vi "Word Search.vi"() -> ()   [LabVIEW 2020]
panel:
  in  "number of words":i32=300
  in  "Max Word Length":u64=150
  in  "Min Word Length":u64=10
  in  "size (rows, columns)":i32[](array[numeric])=[300, 300]
  in  "Solver Selector":T1(radio)
  out "All Words Found":bool
  out "Execution Time":dbl
  # "Use this Test Harness VI to time your Word Search solution (and ensure it works correctly)."
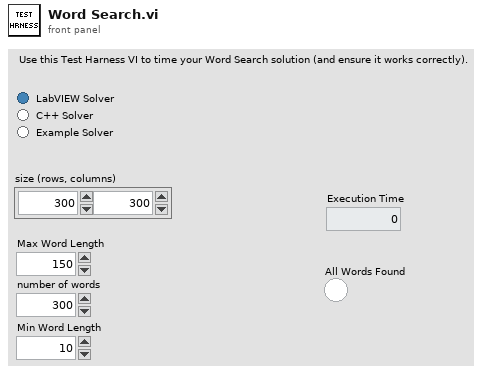
[diagram p1: front panel]
types:
  T1 = enum32{"Your Solver", "C++ Solver", "Example Solver"}
  T2 = typedef "Solutions--map.ctl" = map{string, T3[]}
  T3 = typedef "Letter Index--cluster.ctl" = cluster{"Row":i32, "Column":i32}
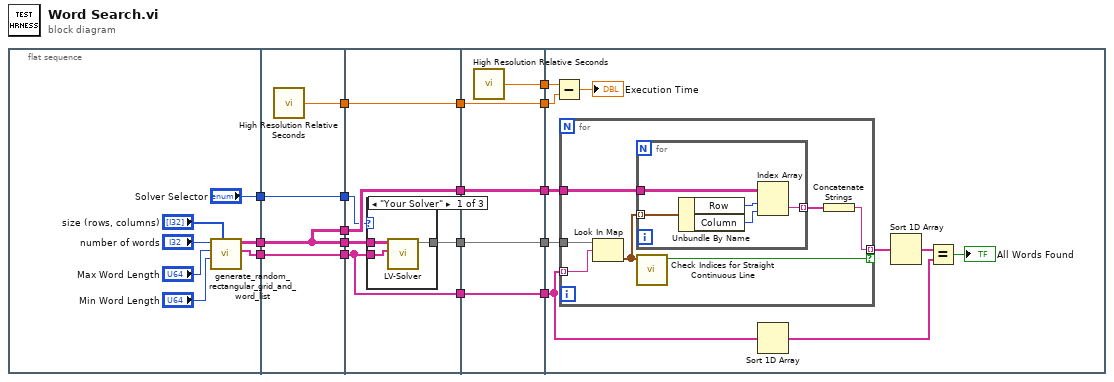
[diagram p0: block diagram]
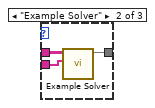
[diagram p2: hidden frame]
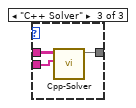
[diagram p3: hidden frame]
diagram:
  n1 = flat-sequence {
    tunnel: [w23] -> w17
    tunnel: [w22] -> w16
    tunnel: ["Solver Selector"] -> w1
    tunnel: w17 -> [w26]
    tunnel: w16 -> [w28]
    tunnel: [w28] -> w15
    tunnel: [w26] -> w14
    tunnel: [w27] -> w10
    tunnel: [w26] -> w3
    tunnel: [w25] -> w2
    tunnel: w1 -> [w25]
    tunnel: w15 -> [w31]
    tunnel: w14 -> [w34]
    tunnel: [w33] -> w13
    tunnel: w10 -> [w32]
    tunnel: [w32] -> w9
    tunnel: [w31] -> w6
    tunnel: [w30] -> w4
    tunnel: w3 -> [w30]
    tunnel: w2 -> [w29]
    tunnel: w13 -> [w48]
    tunnel: [w48] -> w12
    tunnel: [w47] -> w11
    tunnel: w9 -> [w46]
    tunnel: [w46] -> w8
    tunnel: [w45] -> w7
    tunnel: w6 -> [w45]
    tunnel: [w44] -> w5
    tunnel: w4 -> [w44]
    tunnel: w12 -> [w55]
    tunnel: w11 -> [w58]
    tunnel: w8 -> [w57]
    tunnel: w7 -> [w52]
    tunnel: w5 -> [w54]
    frame #0 {
      n2 = call "generate_random_rectangular_grid_and_word_list.vi"("size (rows, columns)"="size (rows, columns)", "Min Word Length"="Min Word Length", "Max Word Length"="Max Word Length", "number of words"="number of words") -> ("Words"=w22:string[], "Grid"=w23:string[][])  [unwired: 6 in]
    }
    frame #1 {
      n3 = call <vilib>:"High Resolution Relative Seconds.vi"() -> ("relative seconds"=w27:dbl)
    }
    frame #2 {
      n4 = case shown="\"Your Solver\"" w29 {
        tunnel: w34 -> [w37 w40 w43]
        tunnel: [w35 w39 w42] -> w33
        tunnel: w31 -> [w36 w38 w41]
        frame "Your Solver" {
          n5 = call "LV-Solver.vi"("Word List"=w36, "Word Search Grid"=w37) -> ("Solutions"=w35:T2)  [unwired: 9 in]
        }
        frame "Example Solver" {
          n6 = call "Example Solver.vi"("Word List"=w38, "Word Search Grid"=w40) -> ("Solutions"=w39:T2)  [unwired: 9 in]
        }
        frame "C++ Solver" {
          n7 = call "Cpp-Solver.vi"("Word List"=w41, "Word Search Grid"=w43) -> ("Solutions"=w42:T2)  [unwired: 9 in]
        }
      }
    }
    frame #3 {
      n8 = call <vilib>:"High Resolution Relative Seconds.vi"() -> ("relative seconds"=w47:dbl)
    }
    frame #4 {
      n9 = Subtract(x=w58, y=w57) -> (x-y=→"Execution Time":dbl)
      n10 = for {
        tunnel: w52 -> [w64] mode=indexing
        tunnel: w55 -> [w65]
        tunnel: w54 -> [w63]
        tunnel: [w61] -> w53 mode=indexing if=w59
        n11 = Look In Map(map=w65, key=w64) -> (value=w60:T3[])  [unwired: 1 in, 1 out]
        n12 = for {
          tunnel: w60 -> [w70] mode=indexing
          tunnel: w63 -> [w68]
          tunnel: [w66] -> w62 mode=indexing
          n13 = Unbundle By Name(w70) -> ("Row"=w69:i32, "Column"=w67:i32)
          n14 = Index Array(array=w68, index (row)=w69, index (col)=w67) -> (element=w66:string)
        }
        n15 = call "Check Indices for Straight Continuous Line.vi"("Letter Indices"=w60) -> ("Straight Continuous Line?"=w59:bool)  [unwired: 10 in]
        n16 = Concatenate Strings(w62) -> (w61:string)
      }
      n17 = Sort 1D Array(array=w52) -> (sorted array=w50:string[])
      n18 = Sort 1D Array(array=w53) -> (sorted array=w51:string[])
      n19 = Equal?(x=w51, y=w50) -> (x = y?=→"All Words Found":bool)
    }
  }
